vi "Analog Encoder Voltage to Angle.vi"(1 "V-min":dbl format="%#_13g", 2 "V-zero":dbl format="%#_13g", 3 "Current Votage":dbl format="%#_13g", 4 "V-max":dbl format="%#_13g") -> (0 "Angle":dbl format="%#_13g")   [LabVIEW 2014]
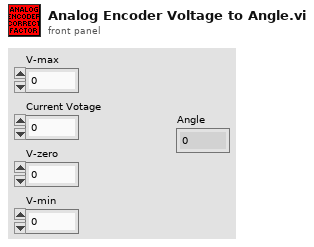
[diagram p1: front panel]
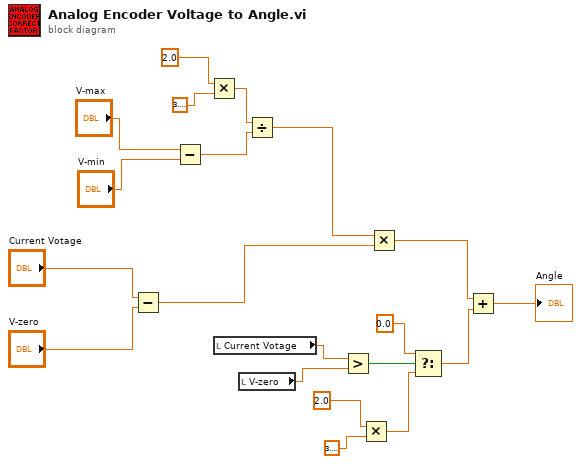
[diagram p0: block diagram]
diagram:
  n1 = Subtract(x="Current Votage", y="V-zero") -> (x-y=w12:dbl)
  n2 = Subtract(x="V-max", y="V-min") -> (x-y=w16:dbl)
  n3 = Multiply(x=2.0, y=3.141592653589793) -> (x*y=w15:dbl)
  n4 = local read "Current Votage"() -> (w10:dbl)
  n5 = local read "V-zero"() -> (w9:dbl)
  n6 = Divide(x=w15, y=w16) -> (x/y=w11:dbl)
  n7 = Greater?(x=w10, y=w9) -> (0:w4:bool)
  n8 = Multiply(x=2.0, y=3.141592653589793) -> (x*y=w3:dbl)
  n9 = Multiply(x=w11, y=w12) -> (x*y=w5:dbl)
  n10 = Select(t=0.0, s=w4, f=w3) -> (s? t:f=w1:dbl)
  n11 = Add(x=w5, y=w1) -> (x+y=→"Angle":dbl)
